vi "FTW-Connector-SpawnNewActor.vi"(0 "FTW Actor Connector Type":refnum<class "FTW-ActorConnector.lvclass">, 5 "Configuration":string="{\n  \"Identity\": \"ActorName\",\n  \"DebugEnableInboxLogging\": false,\n  \"DebugEnableJobLogging\": false,\n  \"InboxAddress\": \"inproc://*\",\n  \"DebugShowPanel\": false\n}", 11 "error in":errorcluster) -> (4 "FTW Actor Connector":refnum<class "FTW-ActorConnector.lvclass">, 6 "Initialized Response":string, 8 "Instance Inbox Address":string, 15 "error out":errorcluster)   [LabVIEW 2013, in "FTW-ActorConnector.lvclass"]
uses:
  FTW-ActorConnector.lvclass
  Endpoint/FTW-Endpoint.lvclass
  JSON/FTW-JSON-Core-LibraryFilepath.vi
  Reflection/FTW-Reflection-Type.vi
  JSON/FTW-JSON-Core-GetFlattenedValue.vi
  JSON/FTW-JSON-Core-LibraryError.vi
  CodeGen/JSON Deserialize/FTW-JSON-Deserialize.xnode
  Ether/FTW-Ether.lvclass
  JSON/FTW-JSON-Native-GetFlattenedValue.vi
  JSON/FTW-JSON-Validate.vi
panel:
  # "Inputs"
  # "Outputs"
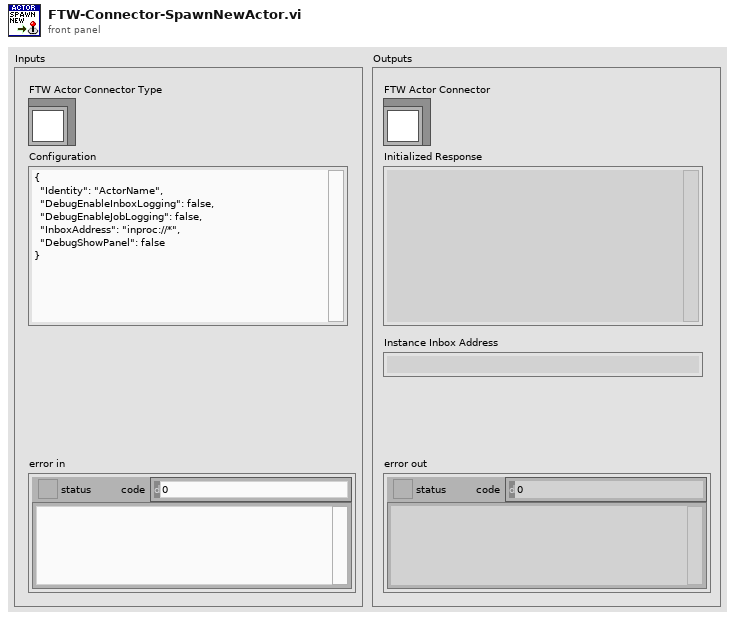
[diagram p1: front panel]
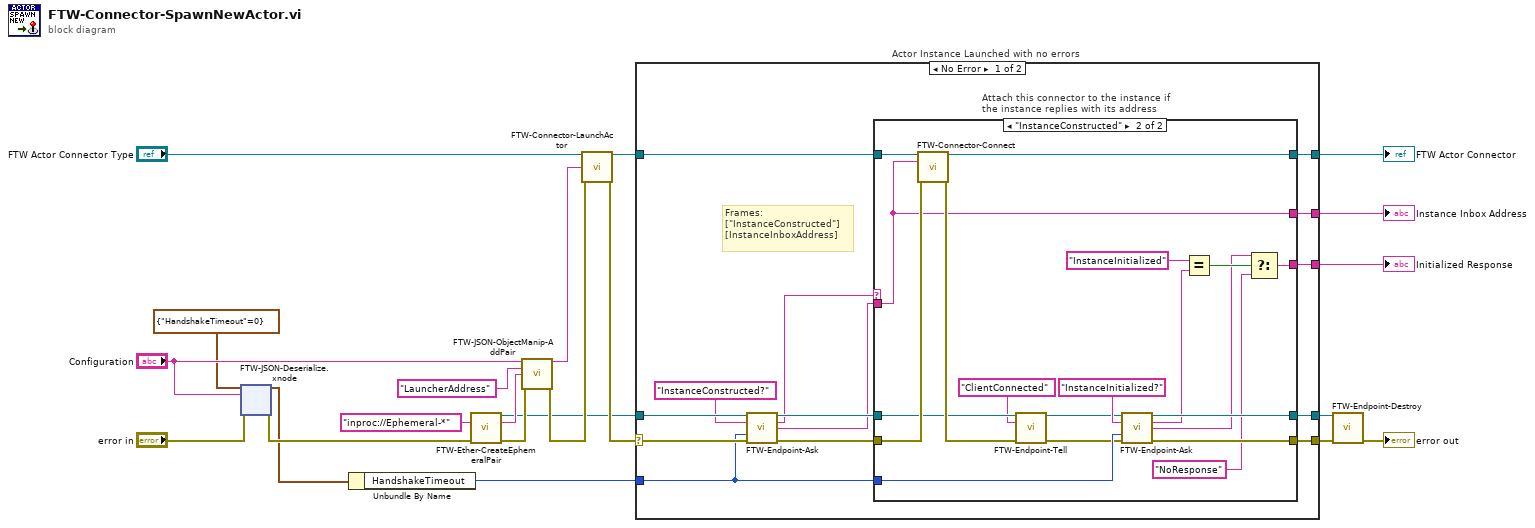
[diagram p0: block diagram]
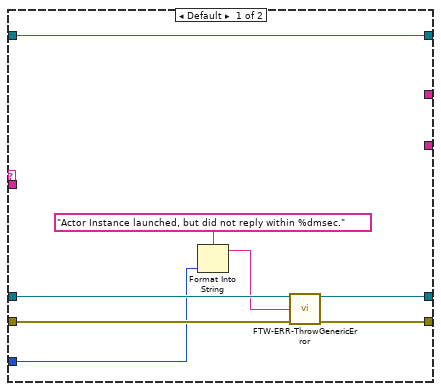
[diagram p2: hidden frame]
diagram:
  n1 = xnode "FTW-JSON-Deserialize.xnode"("Type and Defaults"=cluster{"HandshakeTimeout":i32} {"HandshakeTimeout"=0}, "JSON String"="Configuration", "error in"="error in") -> ("Values"=w3:cluster{"HandshakeTimeout":i32}, "error out"=w22:errorcluster)
  n2 = Unbundle By Name(w3) -> ("HandshakeTimeout"=w2:i32)
  n3 = call "FTW-Ether-CreateEphemeralPair.vi"("Requested Ephemeral Address"="inproc://Ephemeral-*", "error in"=w22) -> ("Ephemeral Endpoint"=w6:refnum<class "FTW-Endpoint.lvclass">, "Actual Ephemeral Address"=w10:string, "error out"=w9:errorcluster)  [unwired: 11 in]
  n4 = call "FTW-JSON-ObjectManip-AddPair.vi"("Input JSON Object"="Configuration", "Key"="LauncherAddress", "Value"=w10, "error in"=w9) -> ("Output JSON Object"=w8:string, "error out"=w12:errorcluster)  [unwired: 10 in]
  n5 = call-dynamic "FTW-Connector-LaunchActor.vi"("FTW Actor Connector Type"="FTW Actor Connector Type", "Configuration"=w8, "error in"=w12) -> ("FTW Actor Connector"=w13:refnum<class "FTW-ActorConnector.lvclass">, "error out"=w11:errorcluster)  [unwired: 11 in]
  n6 = case "Actor Instance Launched with no errors" shown="No Error" w11 {
    selector: w11 -> [w31 w64]
    tunnel: [w36 w64] -> w14
    tunnel: w13 -> [w35 w65]
    tunnel: [w34 w65] -> w20
    tunnel: w6 -> [w32 w63]
    tunnel: w2 -> [w30 _]
    tunnel: [w33 w63] -> w15
    tunnel: [w27 _] -> w18
    tunnel: [w26 _] -> w17
    frame No Error {
      # "Frames:\n[\"InstanceConstructed\"]\n[InstanceInboxAddress]"
      n7 = call-dynamic "FTW-Endpoint-Ask.vi"("FTW Endpoint"=w32, "Request Header"="InstanceConstructed?" ("Header"), "Timeout"=w30, "error in"=w31) -> ("FTW Endpoint out"=w28:refnum<class "FTW-Endpoint.lvclass">, "Response Header"=w24:string, "Response Body"=w23:string, "error out"=w29:errorcluster)  [unwired: 5 in, 3 out]
      n8 = case "Attach this connector to the instance if\nthe instance replies with its address" shown="\"InstanceConstructed\"" w24 {
        tunnel: [w41 w57] -> w36
        tunnel: w35 -> [w43 w60]
        tunnel: [w43 w59] -> w34
        tunnel: w28 -> [w40 w47]
        tunnel: w29 -> [w42 w61]
        tunnel: [w40 w58] -> w33
        tunnel: w30 -> [w38 w49]
        tunnel: w23 -> [_ w48]
        tunnel: [_ w50] -> w27
        tunnel: [_ w48] -> w26
        frame Default {
          n9 = Format Into String(format string="Actor Instance launched, but did not reply within %dmsec." ("Error Message"), w38) -> (resulting string=w37:string)  [unwired: 2 in, 1 out]
          n10 = call "FTW-ERR-ThrowGenericError.vi"("Error Message"=w37, "error in"=w42) -> ("error out"=w41:errorcluster)  [unwired: 13 in]
        }
        frame "InstanceConstructed" {
          n11 = call-dynamic "FTW-Connector-Connect.vi"("FTW Actor Connector Type"=w60, "Instance Inbox Address"=w48, "error in"=w61) -> ("FTW Actor Connector"=w59:refnum<class "FTW-ActorConnector.lvclass">, "error out"=w62:errorcluster)  [unwired: 11 in]
          n12 = call-dynamic "FTW-Endpoint-Tell.vi"("FTW Endpoint"=w47, "Message Header"="ClientConnected", "error in"=w62) -> ("FTW Endpoint out"=w46:refnum<class "FTW-Endpoint.lvclass">, "error out"=w45:errorcluster)  [unwired: 10 in, 1 out]
          n13 = call-dynamic "FTW-Endpoint-Ask.vi"("FTW Endpoint"=w46, "Request Header"="InstanceInitialized?", "Timeout"=w49, "error in"=w45) -> ("FTW Endpoint out"=w58:refnum<class "FTW-Endpoint.lvclass">, "Response Header"=w54:string, "Response Body"=w52:string, "error out"=w57:errorcluster)  [unwired: 5 in, 3 out]
          n14 = Equal?(x="InstanceInitialized", y=w54) -> (x = y?=w53:bool)
          n15 = Select(t=w52, s=w53, f="NoResponse") -> (s? t:f=w50:string)
        }
      }
    }
    frame Error {
    }
  }
  "FTW Actor Connector" <- w20
  "Initialized Response" <- w18
  "Instance Inbox Address" <- w17
  n16 = call-dynamic "FTW-Endpoint-Destroy.vi"("FTW Endpoint"=w15, "error in"=w14) -> ("error out"=→"error out":errorcluster)  [unwired: 13 in]
